vi "AIT 1553 Remote Terminal Page.vi"(8 "error in (no error)":errorcluster, 11 "Node Ptr":T1 format="%.0x") -> (0 "error out":errorcluster)   [LabVIEW 2013]
uses:
  <vilib>/NI Veristand/Custom Device API/Custom Device Item Ref.ctl
  Controls and Global/Global.vi
  <vilib>/NI Veristand/Custom Device API/Get Item Property (U16).vi
  <vilib>/NI Veristand/Custom Device API/Custom Device API.lvlib
  AIT 664 Custom Device.lvlib
panel:
  in  "Read Rate":u16
  in  "Header":cluster{"Section Name":string}={"Section Name"="AIT 1553 Remote Terminal Page"}
  in  "Description":string
  out "Name":string
  # "Hz"
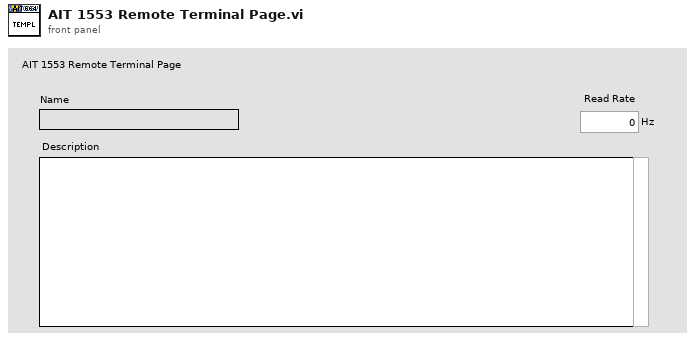
[diagram p1: front panel]
types:
  T1 = typedef "Custom Device API.lvlib/Custom Device Item Ref.ctl" = u64
  T2 = typedef "Custom Device API.lvlib/Custom Device Item Info.ctl" = cluster{"Name":string, "Is Channel":bool, "GUID":string, "Is Waveform":bool}
  T3 = typedef "Custom Device API.lvlib/Custom Device Commands.ctl" = enum16{"Default", "Item renamed", "Shutdown", "Dynamic button pressed"}
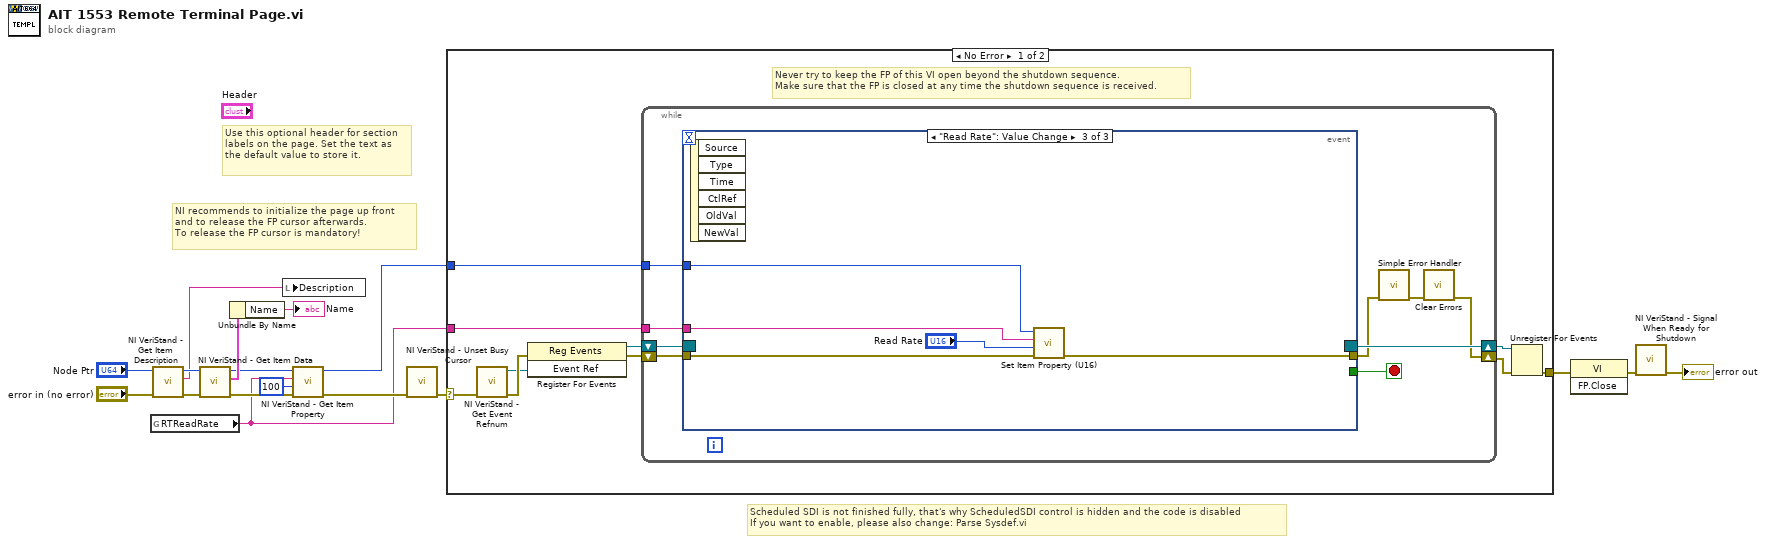
[diagram p0: block diagram]
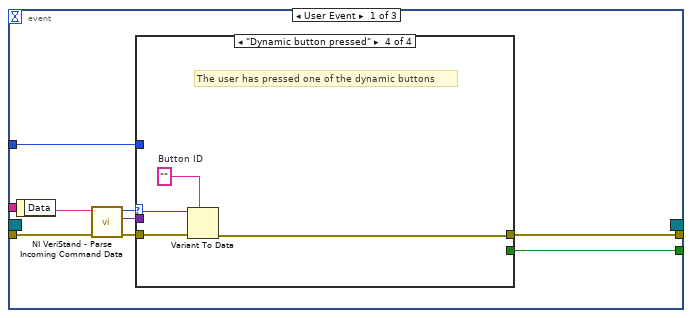
[diagram p2: hidden frame]
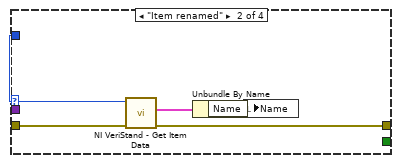
[diagram p4: hidden frame]
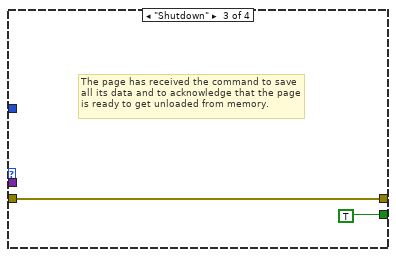
[diagram p5: hidden frame]
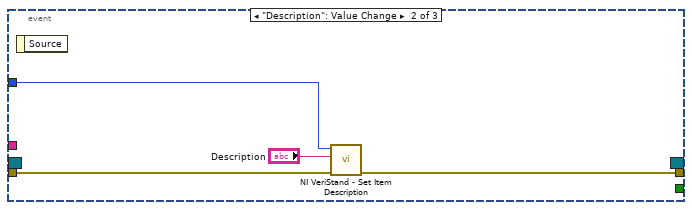
[diagram p6: hidden frame]
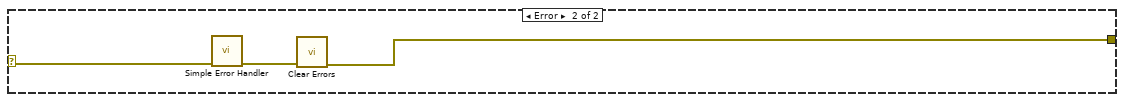
[diagram p7: hidden frame]
diagram:
  # "Scheduled SDI is not finished fully, that's why ScheduledSDI control is hidden and the code is disabled\nIf you want to enable, please also change: Parse Sysdef.vi"
  # "Use this optional header for section labels on the page. Set the text as the default value to store it."
  # "NI recommends to initialize the page up front\nand to release the FP cursor afterwards.\nTo release the FP cursor is mandatory!"
  n1 = global read "Global.vi" "RTReadRate"() -> (w1:string)
  n2 = call <vilib>:"NI VeriStand - Get Item Description.vi"("error in (no error)"="error in (no error)", "Item Ref in"="Node Ptr") -> ("error out"=w11:errorcluster, "Description"=w12:string, "Item Ref out"=w13:T1)  [unwired: 7 out]
  n3 = call <vilib>:"NI VeriStand - Get Item Data.vi"("error in (no error)"=w11, "Item Ref in"=w13) -> ("error out"=w8:errorcluster, "Item Info"=w10:T2, "Item Ref out"=w9:T1)  [unwired: 7 out]
  n4 = Unbundle By Name(w10) -> ("Name"=→"Name":string)
  n5 = local write "Description"(w12) -> ()
  n6 = call-poly <vilib>:"NI VeriStand - Get Item Property.vi"("error in (no error)"=w8, "Default Value"=u16 100, "Property Name"=w1, "Item Ref in"=w9) -> ("error out"=w6:errorcluster, "Item Ref out"=w7:T1)  [unwired: 4 in, 2 out]
  n7 = call <vilib>:"NI VeriStand - Unset Busy Cursor.vi"("error in (no error)"=w6) -> ("error out"=w14:errorcluster)  [unwired: 10 out]
  n8 = case shown="No Error" w14 {
    selector: w14 -> [w19 w68]
    tunnel: [w24 w66] -> w17
    tunnel: w7 -> [w20 _]
    tunnel: w1 -> [w18 _]
    frame No Error {
      # "Never try to keep the FP of this VI open beyond the shutdown sequence.\nMake sure that the FP is closed at any time the shutdown sequence is received."
      n9 = call <vilib>:"NI VeriStand - Get Event Refnum.vi"("error in (no error)"=w19) -> ("error out"=w27:errorcluster, "Event Ref"=w23:refnum<user-event>)  [unwired: 9 out]
      n10 = register-events(error in=w27, w23) -> (reference out=w21:refnum<event-registration>, error out=w22:errorcluster)  [unwired: 1 in]
      n11 = while {
        tunnel: w20 -> [w32]
        shift-right: [w29] -> w25
        shift-left: w22 -> [w35]
        shift-right: [w36] -> w26
        shift-left: w21 -> [w34]
        tunnel: w18 -> [w28]
        stop <- w33 stop-if-true
        n12 = event shown="[2] \"Read Rate\": Value Change" {
          selector: w34 -> [_ _ _]
          dyn-events: [_ _ _] -> w36
          timeout: _ -> [_ _ _]
          tunnel: w35 -> [w44 w59 w65]
          tunnel: [w40 _ _] -> w33
          tunnel: [w39 w58 w64] -> w31
          tunnel: w32 -> [w38 w60 w61]
          tunnel: w28 -> [_ _ w62]
          event User Event {
            n13 = event-data() -> ("Data"=w43:string)  [unwired: 1 out]
            n14 = call <vilib>:"NI VeriStand - Parse Incoming Command Data.vi"("error in (no error)"=w44, "Incoming data"=w43) -> ("error out"=w42:errorcluster, "Outgoing data"=w37:variant, "Action"=w41:T3)  [unwired: 7 out]
            n15 = case shown="\"Dynamic button pressed\"" w41 {
              tunnel: w42 -> [w45 w50 w51 w56]
              tunnel: [_ _ TRUE _] -> w40
              tunnel: [w45 w47 w51 w53] -> w39
              tunnel: w38 -> [_ w49 _ _]
              tunnel: w37 -> [_ _ _ w55]
              frame "Default", Default {
              }
              frame "Item renamed" {
                n16 = call <vilib>:"NI VeriStand - Get Item Data.vi"("error in (no error)"=w50, "Item Ref in"=w49) -> ("error out"=w47:errorcluster, "Item Info"=w48:T2)  [unwired: 8 out]
                n17 = Unbundle By Name(w48) -> ("Name"=w46:string)
                n18 = local write "Name"(w46) -> ()
              }
              frame "Shutdown" {
                # "The page has received the command to save all its data and to acknowledge that the page is ready to get unloaded from memory."
              }
              frame "Dynamic button pressed" {
                w54 = ""  # Button ID
                # "The user has pressed one of the dynamic buttons"
                n19 = Variant To Data(error in=w56, type=w54, Variant=w55) -> (error out=w53:errorcluster)  [unwired: 1 out]
              }
            }
          }
          event "Description": Value Change {
            n20 = event-data() -> ()  [unwired: 2 out]
            n21 = call <vilib>:"NI VeriStand - Set Item Description.vi"("error in (no error)"=w59, "Description"="Description", "Item Ref in"=w60) -> ("error out"=w58:errorcluster)  [unwired: 8 out]
          }
          event "Read Rate": Value Change {
            n22 = event-data() -> ()  [unwired: 7 out]
            n23 = call <vilib>:"Set Item Property (U16).vi"("error in (no error)"=w65, "Value"="Read Rate", "Property Name"=w62, "Item Ref in"=w61) -> ("error out"=w64:errorcluster)  [unwired: 5 in, 2 out]
          }
        }
        n24 = call <vilib>:"Simple Error Handler.vi"("error in (no error)"=w31) -> ("error out"=w30:errorcluster)  [unwired: 1 in, 7 out]
        n25 = call <vilib>:"Clear Errors.vi"("error in (no error)"=w30) -> ("error out"=w29:errorcluster)  [unwired: 6 out]
      }
      n26 = Unregister For Events(event registration refnum=w26, error in=w25) -> (error out=w24:errorcluster)
    }
    frame Error {
      n27 = call <vilib>:"Simple Error Handler.vi"("error in (no error)"=w68) -> ("error out"=w67:errorcluster)  [unwired: 1 in, 7 out]
      n28 = call <vilib>:"Clear Errors.vi"("error in (no error)"=w67) -> ("error out"=w66:errorcluster)  [unwired: 6 out]
    }
  }
  n29 = invoke class="VI" method="FP.Close"(error in=w17) -> (error out=w16:errorcluster)  [unwired: 2 in, 2 out]
  n30 = call <vilib>:"NI VeriStand - Signal When Ready for Shutdown.vi"("error in (no error)"=w16) -> ("error out"=→"error out":errorcluster)  [unwired: 10 out]
